vi "pack_array_len.vi"(3 "error in":errorcluster, 4 "n":u32, 5 "p":u64) -> (0 "error out":errorcluster, 2 "p out":u64)   [LabVIEW 2019, in "msgpack.lvlib"]
doc: "Since msgpack arrays may be heterogeneous, this function packs a header into the buffer that indicates that the following N objects form a single array.\n\nA LabVIEW array can be packed directly using the pack_item VI"
uses:
  msgpack.lvlib
  msgpackalt.dll
panel:
  # "msgpack"
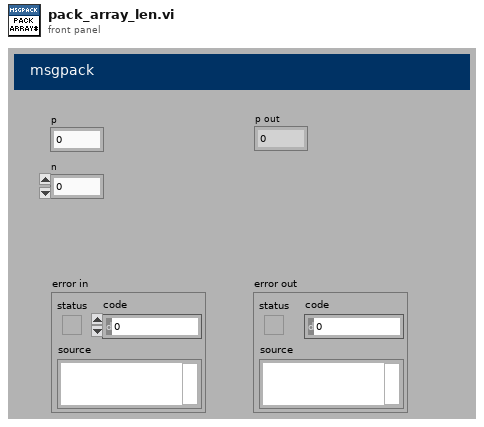
[diagram p1: front panel]
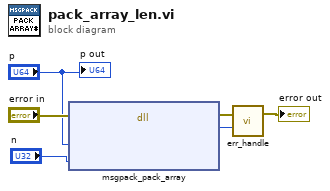
[diagram p0: block diagram]
diagram:
  n1 = dll-call lib="C:/Users/Patrick/Documents/GitHub/Instrument-Framework/lvsrc/SMOs/JSON-RPC-2019/lv-venv/lv.lib/vi.lib/addons/msgpack/msgpackalt.dll" fn="msgpack_pack_array"(error in="error in", "p"="p", "n"="n") -> (error out=w3:errorcluster, "return type"=w4:i32)  [unwired: 4 in, 1 out]
  n2 = call "err_handle.vi"("retval"=w4, "error in"=w3) -> ("error out"=→"error out":errorcluster)  [unwired: 1 in]
  "p out" <- "p"
